vi "Get All Headers.vi"(8 "error in (no error)":errorcluster, 11 "REST Client Headers_NET in":refnum<class "REST Client Headers_NET.lvclass">) -> (0 "error out":errorcluster, 1 "Values":string[](array[string]), 2 "Names":string[](array[string]), 3 "REST Client Headers_NET out":refnum<class "REST Client Headers_NET.lvclass">)   [LabVIEW 2018, in "REST Client_NET.lvlib" / "REST Client Headers_NET.lvclass"]
doc: "Get all HTTP response hader names and corresponding values.\n<b> </b> <b> </b>\nHttpClient_NET\nJustin Young - Viviota\nCopyright (c) 2021\nLicense: BSD"
uses:
  REST Client Headers_NET.lvclass
  REST Client Headers_NET.lvclass/REST Client Headers_NET.ctl
  HttpHeaders_content/HttpHeaders_Content.lvclass
  C:/Viviota/Projects/R&D/LabVIEW_HTTP_REST_NET/HTTPHeaders_NET/HttpHeaders_NET.lvclass
  HttpHeaders_response/HttpHeaders_Response.lvclass
  HTTPHeaders_NET/HttpHeaders_NET.lvclass
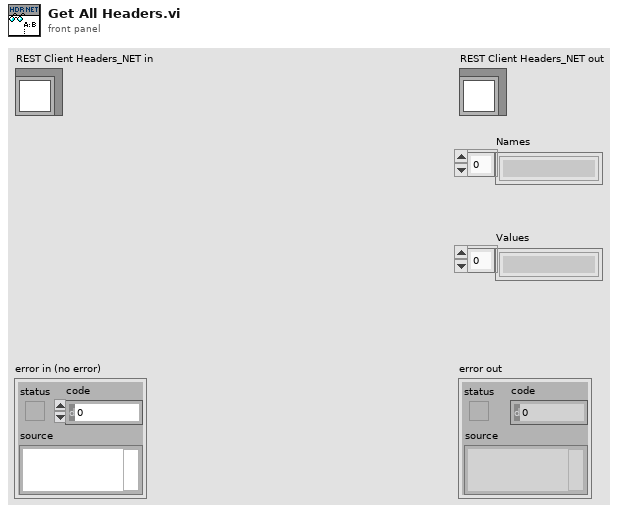
[diagram p1: front panel]
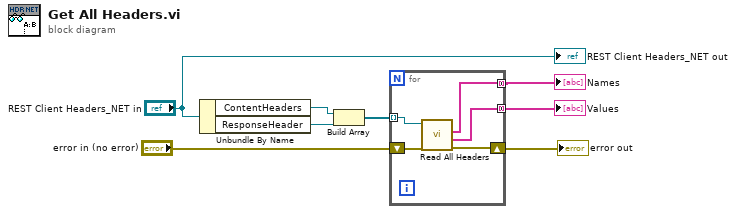
[diagram p0: block diagram]
diagram:
  n1 = Unbundle By Name("REST Client Headers_NET in") -> ("ContentHeaders"=w6:refnum<class "HttpHeaders_Content.lvclass">, "ResponseHeader"=w7:refnum<class "HttpHeaders_Response.lvclass">)
  n2 = Build Array(w6, w7) -> (w4:refnum<class "HttpHeaders_NET.lvclass">[])
  n3 = for {
    shift-right: [w11] -> w1
    shift-left: "error in (no error)" -> [w13]
    tunnel: w4 -> [w12] mode=indexing
    tunnel: [w10] -> w3 mode=concatenating
    tunnel: [w9] -> w2 mode=concatenating
    n4 = call-dynamic "Read All Headers.vi"("error in (no error)"=w13, "HTTPHeaders_NET in"=w12) -> ("error out"=w11:errorcluster, "Header Values"=w9:string[], "Header Names"=w10:string[])  [unwired: 6 in, 1 out]
  }
  "error out" <- w1
  "Names" <- w3
  "Values" <- w2
  "REST Client Headers_NET out" <- "REST Client Headers_NET in"
